vi "NeedleValveClose - Encoder.vi"(8 "error in (no error)":errorcluster, 10 "Percent Difference":i32, 11 "VISA resource name":refnum<visa-resource-name>) -> (0 "error out":errorcluster, 3 "VISA resource name out":refnum<visa-resource-name>)   [LabVIEW 2018]
uses:
  Request.ctl
  ZaberTSeries.lvlib
panel:
  out "data":dbl
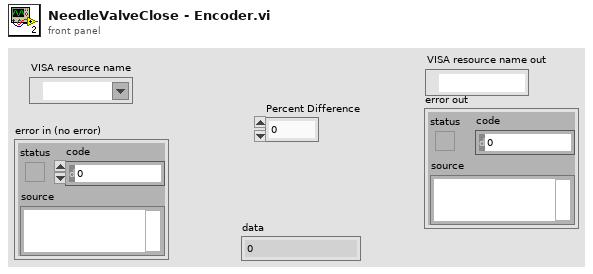
[diagram p1: front panel]
types:
  T1 = typedef "ZaberTSeries.lvlib/Request.ctl" = cluster{"Device Number":u8, "Command":u8, "Data":i32, "Response Count":i32}
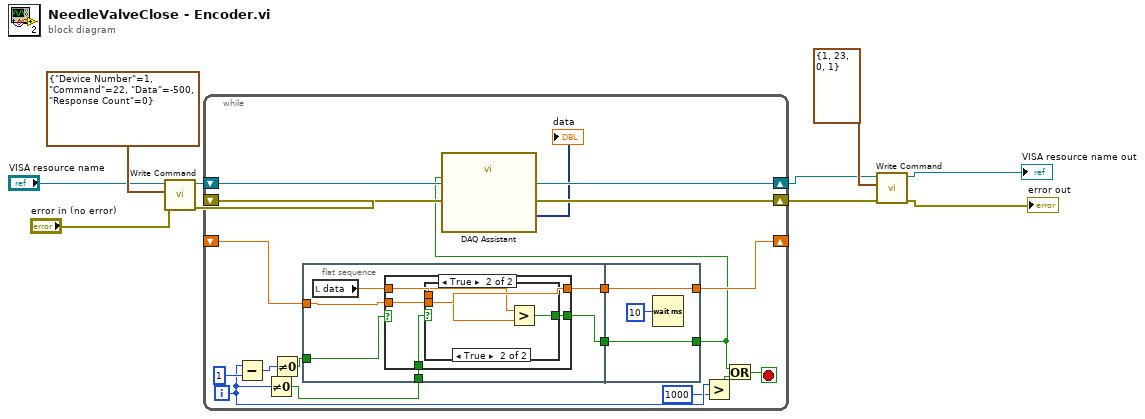
[diagram p0: block diagram]
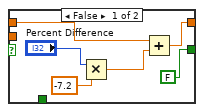
[diagram p2: hidden frame]
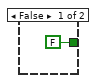
[diagram p3: hidden frame]
diagram:
  n1 = call "Write Command.vi"("error in (no error)"="error in (no error)", "Request"=T1 {"Device Number"=1, "Command"=22, "Data"=-500, "Response Count"=0}, "VISA resource name"="VISA resource name") -> ("error out"=w8:errorcluster, "VISA resource name out"=w9:refnum<visa-resource-name>)  [unwired: 6 in, 1 out]
  n2 = while {
    shift-right: [w26] -> w4
    shift-left: w9 -> [w26]
    shift-right: [w25] -> w2
    shift-left: w8 -> [w25]
    shift-right: [w20] -> _
    shift-left: _ -> [w19]
    i -> [w12]
    stop <- w14 stop-if-true
    n3 = Subtract(x=w12, y=1) -> (x-y=w17:i32)
    n4 = Not Equal To 0?(x=w12) -> (x != 0?=w16:bool)
    n5 = Not Equal To 0?(x=w17) -> (x != 0?=w22:bool)
    n6 = flat-sequence {
      tunnel: [w31] -> w23
      tunnel: w22 -> [w30]
      tunnel: [w29] -> w21
      tunnel: w19 -> [w28]
      tunnel: w16 -> [w27]
      tunnel: [w49] -> w15
      tunnel: w23 -> [w49]
      tunnel: [w47] -> w20
      tunnel: w21 -> [w47]
      frame #0 {
        n7 = local read "data"() -> (w32:dbl)
        n8 = case shown="True" w30 {
          tunnel: w32 -> [w35 w42]
          tunnel: [FALSE w41] -> w31
          tunnel: [w34 w40] -> w29
          tunnel: w28 -> [_ w40]
          tunnel: w27 -> [_ w39]
          frame False {
            n9 = Multiply(x="Percent Difference", y=-7.2) -> (x*y=w36:dbl)
            n10 = Add(x=w35, y=w36) -> (x+y=w34:dbl)
          }
          frame True {
            n11 = case shown="True" w39 {
              tunnel: w42 -> [_ w46]
              tunnel: [FALSE w45] -> w41
              tunnel: w40 -> [_ w44]
              frame False {
              }
              frame True {
                n12 = Greater?(x=w46, y=w44) -> (0:w45:bool)
              }
            }
          }
        }
      }
      frame #1 {
        n13 = Wait (ms)(milliseconds to wait=u32 10) -> ()  [unwired: 1 out]
      }
    }
    n14 = call "DAQ Assistant"("stop (F)"=w15) -> ("data"=→"data":dynamicdata)  [unwired: 15 in, 3 out]
    n15 = Greater?(x=w12, y=1000) -> (0:w13:bool)
    n16 = Or(x=w15, y=w13) -> (x .or. y?=w14:bool)
  }
  n17 = call "Write Command.vi"("error in (no error)"=w2, "Request"=T1 {"Device Number"=1, "Command"=23, "Data"=0, "Response Count"=1}, "VISA resource name"=w4) -> ("error out"=→"error out":errorcluster, "VISA resource name out"=→"VISA resource name out":refnum<visa-resource-name>)  [unwired: 6 in, 1 out]
